vi "RSZVB Delete Memory Trace.vi"(8 "error in (no error)":errorcluster {"code" format="%.0x"}, 10 "Memory Trace (0: Memory Trace 1)":i32(ring) items=["Memory Trace 1", "Memory Trace 2", "Memory Trace 3", "Memory Trace 4", "Memory Trace 5", "Memory Trace 6", "Memory Trace 7", "Memory Trace 8"], 11 "VISA session":refnum<visa-resource-name>) -> (0 "error out":errorcluster {"code" format="%.0x"}, 3 "dup VISA session":refnum<visa-resource-name>)   [LabVIEW 2011]
doc: "This VI deletes one of the memory traces Mem<n>[Trc<m>], where n = 1, ... 8.\n\nRemote-control command(s):\nTRACe:CLEar MDATA1 | MDATA2 | MDATA3 | MDATA4 | MDATA5 | MDATA6 | MDATA7 | MDATA8"
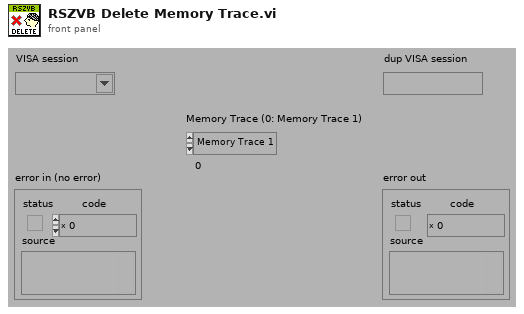
[diagram p1: front panel]
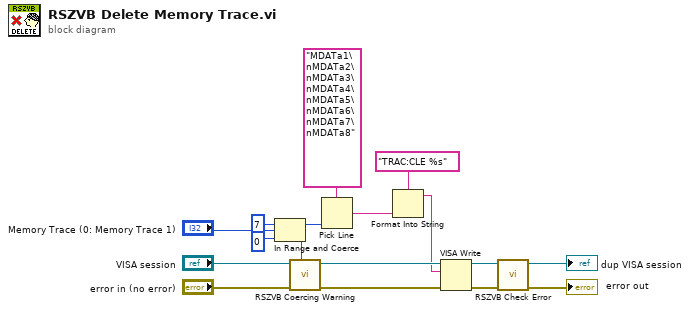
[diagram p0: block diagram]
diagram:
  n1 = In Range and Coerce(upper limit=7, x="Memory Trace (0: Memory Trace 1)", lower limit=0) -> (coerced(x)=w10:i32, In Range?=w6:bool)
  n2 = call "RSZVB Coercing Warning.vi"("In Range?"=w6, "error in (no error)"="error in (no error)", "VISA session"="VISA session") -> ("error out"=w15:errorcluster, "dup VISA session"=w16:refnum<visa-resource-name>)  [unwired: 7 in]
  n3 = Pick Line(multi-line string="MDATa1\nMDATa2\nMDATa3\nMDATa4\nMDATa5\nMDATa6\nMDATa7\nMDATa8", line index=w10) -> (output string=w11:string)  [unwired: 1 in]
  n4 = Format Into String(format string="TRAC:CLE %s", w11) -> (resulting string=w12:string)  [unwired: 2 in, 1 out]
  n5 = VISA Write(VISA resource name=w16, write buffer=w12, error in (no error)=w15) -> (VISA resource name out=w13:refnum<visa-resource-name>, error out=w14:errorcluster)  [unwired: 1 out]
  n6 = call "RSZVB Check Error.vi"("error in (no error)"=w14, "VISA session"=w13) -> ("error out"=→"error out":errorcluster, "dup VISA session"=→"dup VISA session":refnum<visa-resource-name>)  [unwired: 8 in]
